vi "Test.vi"() -> ()   [LabVIEW 2017]
doc: "This VI is called when test mode begins, and will automatically be terminated when it ends. You can add manual or automatic tests and invoke them from the dashboard."
panel:
  in  "Tab Control":enum32{"Lift1", "Arm", "Claw Rotation"}(tab)
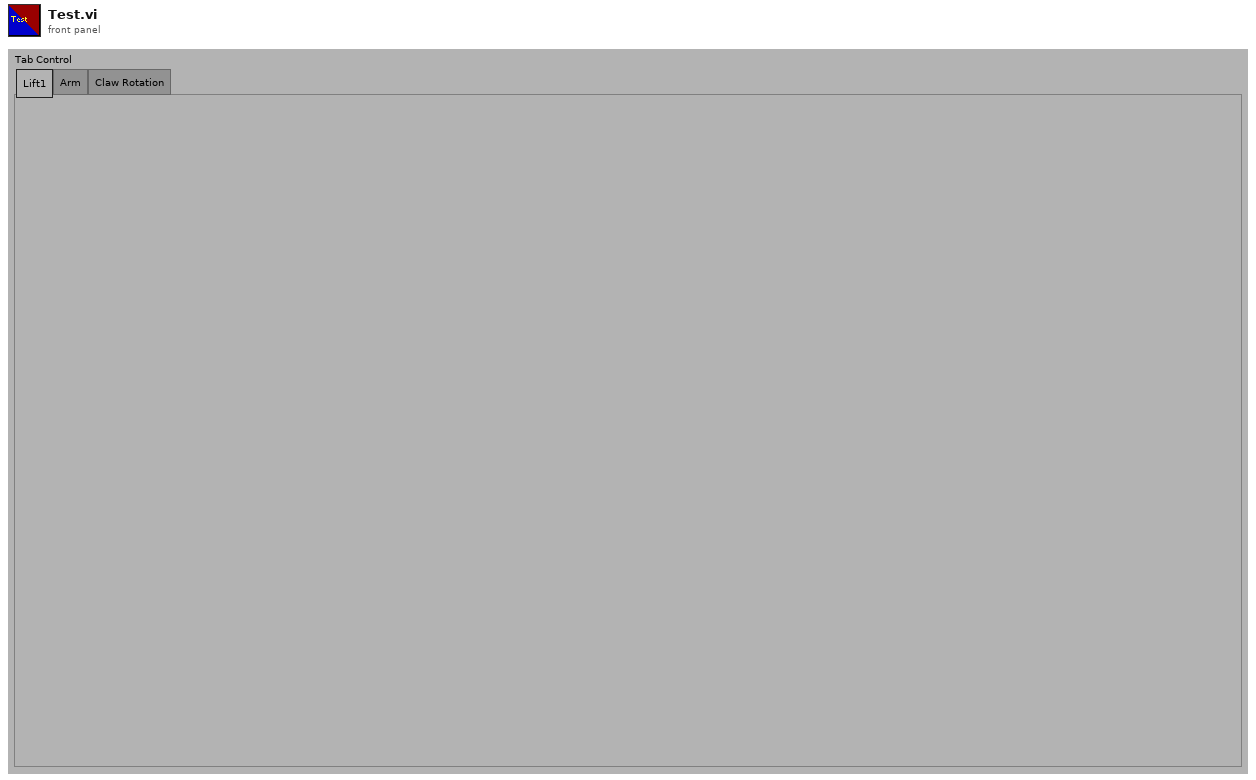
[diagram p1: front panel]
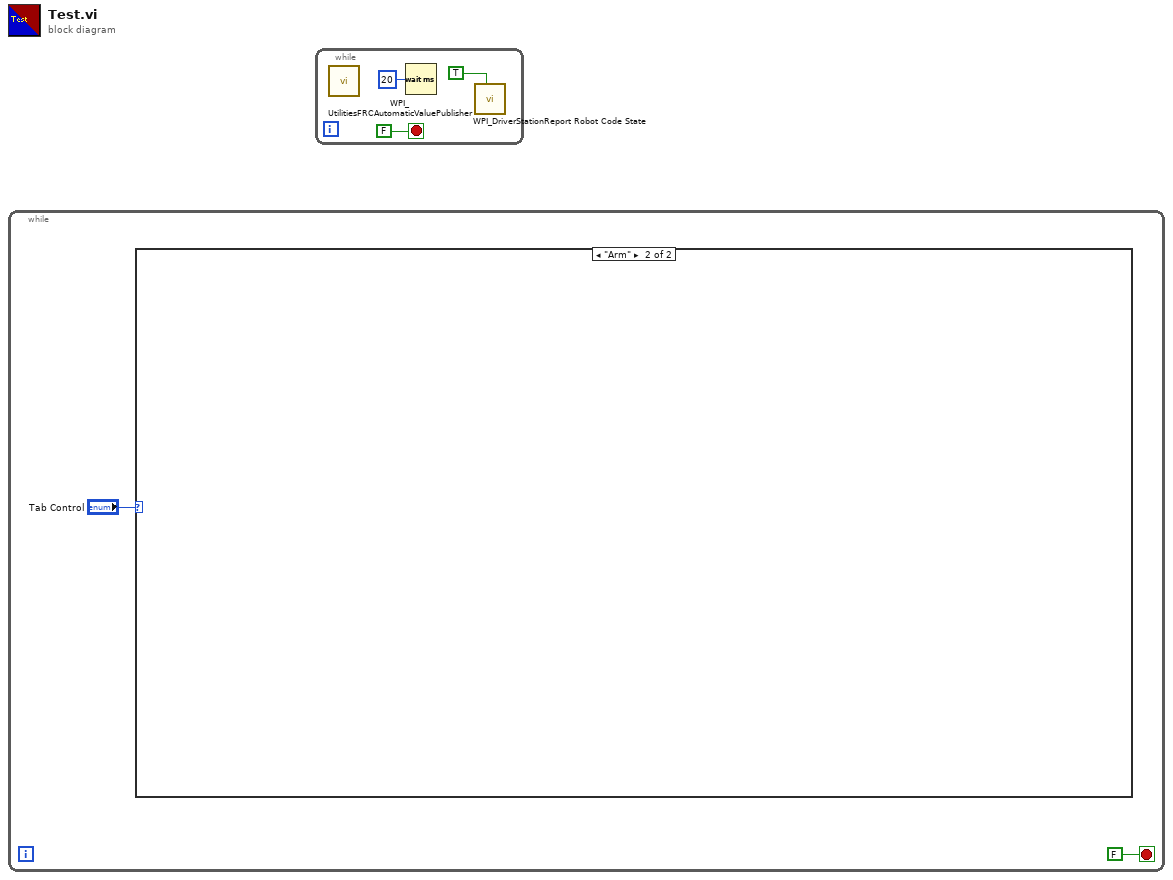
[diagram p0: block diagram]
diagram:
  n1 = while {
    stop <- FALSE stop-if-true
    n2 = case shown="\"Arm\"" "Tab Control" {
      frame "Lift1", Default {
      }
      frame "Arm" {
      }
    }
  }
  n3 = while {
    stop <- FALSE stop-if-true
    n4 = call <vilib>:"WPI_UtilitiesFRCAutomaticValuePublisher.vi"() -> ()  [unwired: 12 in]
    n5 = Wait (ms)(milliseconds to wait=u32 20) -> ()  [unwired: 1 out]
    n6 = call <vilib>:"WPI_DriverStationReport Robot Code State.vi"("Test"=TRUE ("Autonomous")) -> ()  [unwired: 10 in, 1 out]
  }
